vi "Moving Average (multiple).vi"(6 "Window Unit (points)":enum16{"Points", "Data"}(ring), 8 "error in (no error)":errorcluster, 10 "Window":dbl, 11 "XY-data":cluster{"X-array":dbl[], "Y-array":dbl[]}[](array[cluster])) -> (0 "error out":errorcluster, 3 "XY-data out":cluster{"X-array":dbl[], "Y-array":dbl[]}[](array[cluster]) {"Y-array" format="%.2p"; "X-array" format="%.2p"})   [LabVIEW 2019, in "xy_utilities.lvlib"]
doc: "Apply a moving average <b>XY-data</b>'s Y-Array according to <b>window</b>\n\nWire data to the data input to determine the polymorphic instance to use or manually select the instance."
uses:
  xy_utilities.lvlib
  Get Size (multiple).vi
  Get Size (single).vi
  Private/X Array Range to Index.vi
  Get X and Y.vi
  Get X and Y (single).vi
  Circular Buffer (multiple).vi
  <vilib>/ptbypt/NI_PtbyPt.lvlib
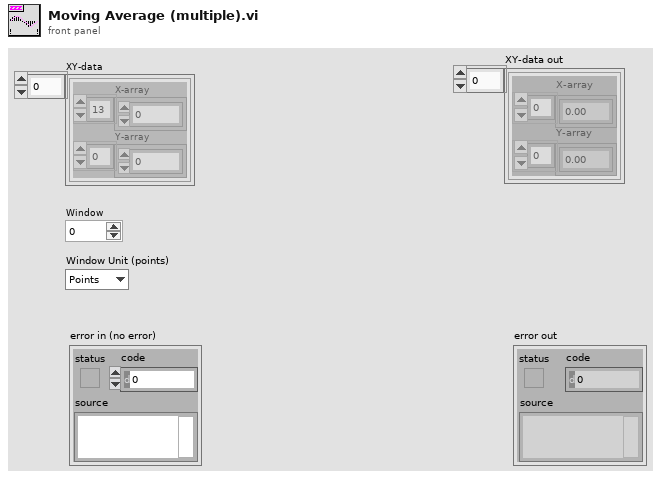
[diagram p1: front panel]
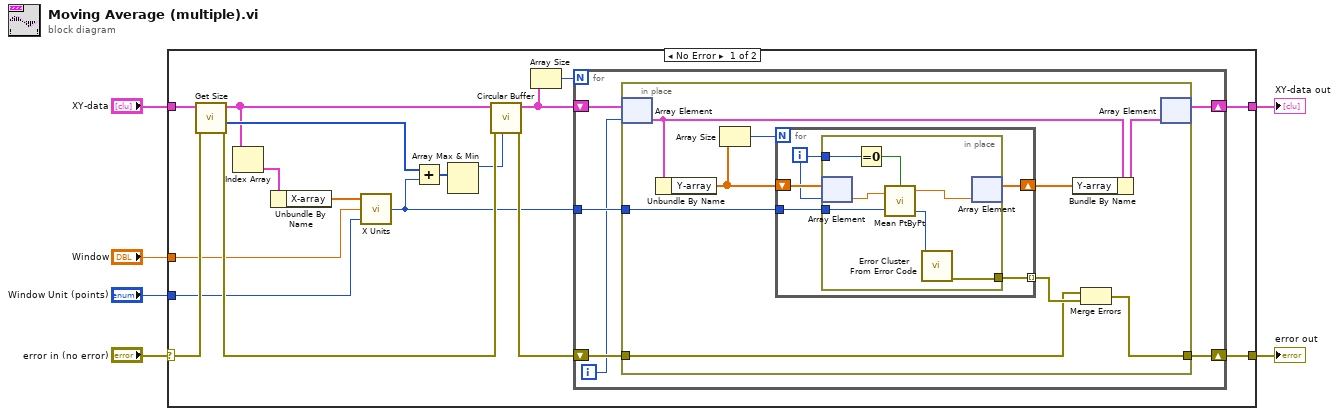
[diagram p0: block diagram]
diagram:
  n1 = case shown="No Error" "error in (no error)" {
    selector: "error in (no error)" -> [w18 w52]
    tunnel: [w12 w52] -> w5
    tunnel: "XY-data" -> [w17 w51]
    tunnel: [w9 w51] -> w3
    tunnel: "Window" -> [w14 _]
    tunnel: "Window Unit (points)" -> [w13 _]
    frame No Error {
      n2 = call-poly "Get Size.vi"("error in (no error)"=w18, "XY-data"=w17) -> ("error out"=w22:errorcluster, "X size"=w19:i32[], "XY-data out"=w11:cluster{"X-array":dbl[], "Y-array":dbl[]}[])  [unwired: 6 in, 1 out]
      n3 = Index Array(array=w11) -> (element=w10:cluster{"X-array":dbl[], "Y-array":dbl[]})  [unwired: 1 in]
      n4 = Unbundle By Name(w10) -> ("X-array"=w23:dbl[])
      n5 = call "X Units.vi"("Interval Units (points)"=w13, "Interval (h)"=w14, "X-array"=w23) -> ("h (points)"=w20:i32)
      n6 = Add(x=w19, y=w20) -> (x+y=w16:i32[])
      n7 = Array Max & Min(array=w16) -> (max value=w15:i32)  [unwired: 3 out]
      n8 = call-poly "Circular Buffer.vi"("History Length [1024]"=w15, "error in"=w22, "XY-data"=w11) -> ("error out"=w21:errorcluster, "XY-data out"=w7:cluster{"X-array":dbl[], "Y-array":dbl[]}[])  [unwired: 7 in]
      n9 = Array Size(array=w7) -> (size(s)=w8:i32)
      n10 = for {
        N: w8 -> [_]
        tunnel: w20 -> [w28]
        shift-right: [w27] -> w12
        shift-left: w21 -> [w29]
        shift-right: [w25] -> w9
        shift-left: w7 -> [w26]
        i -> [w24]
        n11 = in-place {
          in-place-border: w29 -> [w36]
          in-place-border: w28 -> [w35]
          in-place-border: [w34] -> w27
          n12 = in-place-array #1(w26, w24) -> (w33:cluster{"X-array":dbl[], "Y-array":dbl[]})
          n13 = Unbundle By Name(w33) -> ("Y-array"=w30:dbl[])
          n14 = Array Size(array=w30) -> (size(s)=w31:i32)
          n15 = for {
            N: w31 -> [_]
            tunnel: w35 -> [w43]
            tunnel: [w42] -> w37 mode=indexing
            shift-right: [w39] -> w38
            shift-left: w30 -> [w41]
            i -> [w40]
            n16 = in-place {
              in-place-border: w43 -> [w50]
              in-place-border: w40 -> [w48]
              in-place-border: [w46] -> w42
              n17 = in-place-array #2(w41, w40) -> (w45:dbl)
              n18 = Equal To 0?(x=w48) -> (x = 0?=w49:bool)
              n19 = call <vilib>:"Mean PtByPt.vi"("x"=w45, "sample length"=w50, "initialize"=w49) -> ("mean"=w44:dbl, "error"=w47:i32)  [unwired: 1 in]
              n20 = call <vilib>:"Error Cluster From Error Code.vi"("error code (0)"=w47) -> ("error out"=w46:errorcluster)  [unwired: 8 in]
              n21 = in-place-array #2(w44) -> (w39:dbl[])  [unwired: 1 out]
            }
          }
          n22 = Bundle By Name(cluster=w33, "Y-array"=w38) -> (w32:cluster{"X-array":dbl[], "Y-array":dbl[]})
          n23 = Merge Errors(w36, w37) -> (w34:errorcluster)
          n24 = in-place-array #1(w32) -> (w25:cluster{"X-array":dbl[], "Y-array":dbl[]}[])  [unwired: 1 out]
        }
      }
    }
    frame Error {
    }
  }
  "error out" <- w5
  "XY-data out" <- w3
